vi "destan.vi"(1 "variablearray":T1(array[cluster])=[{"ling.var."="in1", "x-min"=-1.0, "x-max"=1.0, "setarray"=[{"linguistic term"="NE1", "color"=0, "points"=[-1.0, -1.0000001192092896, -1.0000001192092896, 0.0]}, {"linguistic term"="ZE1", "color"=0, "points"=[-1.0000001192092896, 0.0, 0.0, 1.0000001192092896]}, {"linguistic term"="PO1", "color"=0, "points"=[1.4901161193847656e-08, 1.0, 1.0, 1.0000001192092896]}]}, {"ling.var."="in2", "x-min"=-1.0, "x-max"=1.0, "setarray"=[{"linguistic term"="NE2", "color"=0, "points"=[-1.0, -1.0000001192092896, -1.0000001192092896, 0.0]}, {"linguistic term"="ZE2", "color"=0, "points"=[-1.0000001192092896, 0.0, 0.0, 1.0000001192092896]}, {"linguistic term"="PO2", "color"=0, "points"=[1.4901161193847656e-08, 1.0, 1.0, 1.0000001192092896]}]}, {"ling.var."="in3", "x-min"=-1.0, "x-max"=1.0, "setarray"=[{"linguistic term"="NE3", "color"=0, "points"=[-1.0, -1.0000001192092896, -1.0000001192092896, 0.0]}, {"linguistic term"="ZE3", "color"=0, "points"=[-1.0000001192092896, 0.0, 0.0, 1.0000001192092896]}, {"linguistic term"="PO3", "color"=0, "points"=[1.4901161193847656e-08, 1.0, 1.0, 1.0000001192092896]}]}, {"ling.var."="in4", "x-min"=-1.0, "x-max"=1.0, "setarray"=[{"linguistic term"="NE4", "color"=0, "points"=[-1.0, -1.0000001192092896, -1.0000001192092896, 0.0]}, {"linguistic term"="ZE4", "color"=0, "points"=[-1.0000001192092896, 0.0, 0.0, 1.0000001192092896]}, {"linguistic term"="PO4", "color"=0, "points"=[1.4901161193847656e-08, 1.0, 1.0, 1.0000001192092896]}]}] {"x-min" format="%.2f"; "x-max" format="%.2f"; "setarray"."points" min=-1.0 max=1.0 step=0.10000000149011612 format="%.2f"}) -> (0 "destandarized variable array":T1(array[cluster])=[{"ling.var."="in1", "x-min"=-1.0, "x-max"=1.0, "setarray"=[{"linguistic term"="NE1", "color"=0, "points"=[-1.0, -1.0000001192092896, -1.0000001192092896, 0.0]}, {"linguistic term"="ZE1", "color"=0, "points"=[-1.0000001192092896, 0.0, 0.0, 1.0000001192092896]}, {"linguistic term"="PO1", "color"=0, "points"=[1.4901161193847656e-08, 1.0, 1.0, 1.0000001192092896]}]}, {"ling.var."="in2", "x-min"=-1.0, "x-max"=1.0, "setarray"=[{"linguistic term"="NE2", "color"=0, "points"=[-1.0, -1.0000001192092896, -1.0000001192092896, 0.0]}, {"linguistic term"="ZE2", "color"=0, "points"=[-1.0000001192092896, 0.0, 0.0, 1.0000001192092896]}, {"linguistic term"="PO2", "color"=0, "points"=[1.4901161193847656e-08, 1.0, 1.0, 1.0000001192092896]}]}, {"ling.var."="in3", "x-min"=-1.0, "x-max"=1.0, "setarray"=[{"linguistic term"="NE3", "color"=0, "points"=[-1.0, -1.0000001192092896, -1.0000001192092896, 0.0]}, {"linguistic term"="ZE3", "color"=0, "points"=[-1.0000001192092896, 0.0, 0.0, 1.0000001192092896]}, {"linguistic term"="PO3", "color"=0, "points"=[1.4901161193847656e-08, 1.0, 1.0, 1.0000001192092896]}]}, {"ling.var."="in4", "x-min"=-1.0, "x-max"=1.0, "setarray"=[{"linguistic term"="NE4", "color"=0, "points"=[-1.0, -1.0000001192092896, -1.0000001192092896, 0.0]}, {"linguistic term"="ZE4", "color"=0, "points"=[-1.0000001192092896, 0.0, 0.0, 1.0000001192092896]}, {"linguistic term"="PO4", "color"=0, "points"=[1.4901161193847656e-08, 1.0, 1.0, 1.0000001192092896]}]}] {"x-min" format="%.2f"; "x-max" format="%.2f"; "setarray"."points" min=-1.0 max=1.0 step=0.10000000149011612 format="%.2f"})   [LabVIEW 2020, in "NI_fuzzy logic.lvlib"]
doc: "VI to destandarise the setpoints of the consequence- or antecedancevariables.\nThe terms are spreaded to the range of the given Minimum and Maximum of each variable."
uses:
  <vilib>/addons/control/fuzzy/NI_fuzzy logic.lvlib
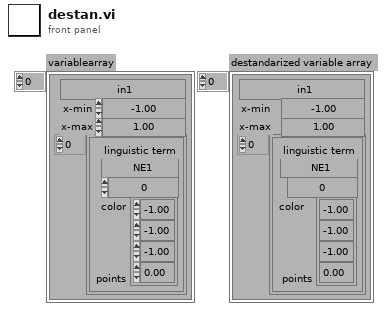
[diagram p1: front panel]
types:
  T1 = cluster{"ling.var.":string, "x-min":dbl, "x-max":dbl, "setarray":cluster{"linguistic term":string, "color":u32, "points":dbl[]}[]}[]
  T2 = cluster{"linguistic term":string, "color":u32, "points":dbl[]}[]
  T3 = cluster{"linguistic term":string, "color":u32, "points":dbl[]}
  T4 = cluster{"ling.var.":string, "x-min":dbl, "x-max":dbl, "setarray":cluster{"linguistic term":string, "color":u32, "points":dbl[]}[]}
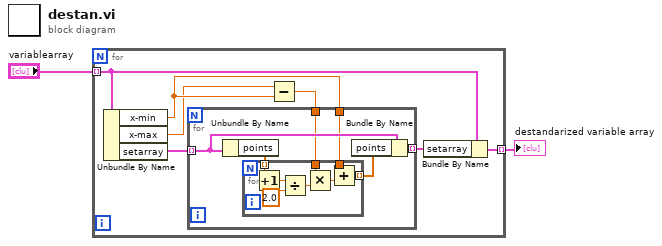
[diagram p0: block diagram]
diagram:
  n1 = for {
    tunnel: "variablearray" -> [w8] mode=indexing
    tunnel: [w9] -> w1 mode=indexing
    n2 = Unbundle By Name(w8) -> ("x-min"=w4:dbl, "x-max"=w3:dbl, "setarray"=w7:T2)
    n3 = Subtract(x=w3, y=w4) -> (x-y=w5:dbl)
    n4 = for {
      tunnel: w7 -> [w15] mode=indexing
      tunnel: [w14] -> w6 mode=indexing
      tunnel: w5 -> [w13]
      tunnel: w4 -> [w12]
      n5 = Unbundle By Name(w15) -> ("points"=w11:dbl[])
      n6 = for {
        tunnel: w11 -> [w23] mode=indexing
        tunnel: w13 -> [w19]
        tunnel: w12 -> [w17]
        tunnel: [w16] -> w10 mode=indexing
        n7 = Increment(x=w23) -> (x+1=w22:dbl)
        n8 = Divide(x=w22, y=2.0) -> (x/y=w20:dbl)
        n9 = Multiply(x=w19, y=w20) -> (x*y=w18:dbl)
        n10 = Add(x=w17, y=w18) -> (x+y=w16:dbl)
      }
      n11 = Bundle By Name(cluster=w15, "points"=w10) -> (w14:T3)
    }
    n12 = Bundle By Name(cluster=w8, "setarray"=w6) -> (w9:T4)
  }
  "destandarized variable array" <- w1
